vi "Generate Sound.vi"() -> ()   [LabVIEW 2017]
doc: "本VI说明了生成并播放正弦波、方波、锯齿波和三角波的方式。在连续播放时可更改生成波形的频率和类型。"
uses:
  <vilib>/sound2/lvsound2.llb/Sampling Mode.ctl
  <vilib>/sound2/lvsound2.llb/Sound Data Format.ctl
  <vilib>/sound2/lvsound2.llb/Sound Output Set Volume (Single).vi
  <vilib>/sound2/lvsound2.llb/Sound Output Write (DBL Single).vi
panel:
  in  "音量":dbl(slide)=50.0 scale=0.0..100.0
  out "生成声音":waveform(dbl)(graph)
  in  "频率":dbl=500.0
  in  "停止":bool
  in  "设备ID":u32
  # "概述：演示使用声音函数连续生成和播放正弦波形。\n操作步骤：\n1.指定设备ID的值。\n2. 运行VI。生成波形并将其发送至图形和扬声器。\n3.修改声音的频率和音量。\n4.单击停止按钮停止VI。"
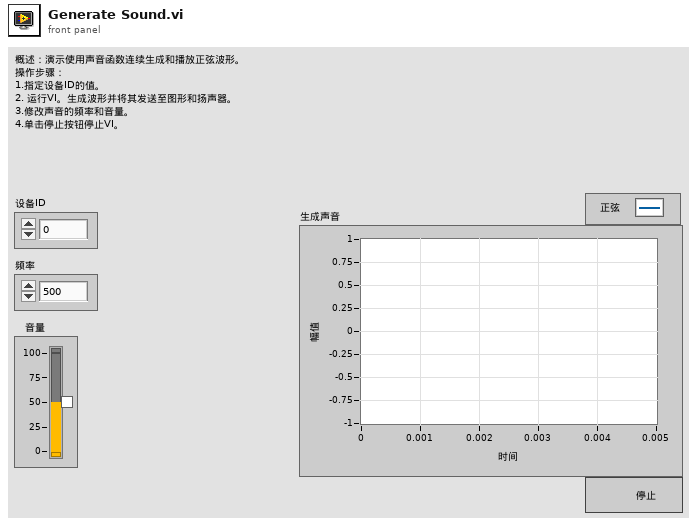
[diagram p1: front panel]
types:
  T1 = typedef "Sound Data Format.ctl" = cluster{"sample rate (S/s)":dbl, "number of channels":i32, "bits per sample":i32}
  T2 = typedef "Sampling Mode.ctl" = i32
  T3 = typedef "Sound Output Task ID.ctl" = u32
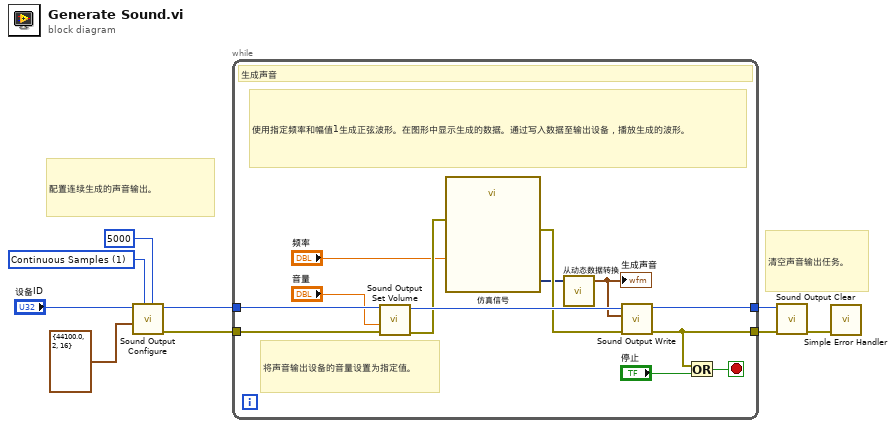
[diagram p0: block diagram]
diagram:
  w4 = T2 1 items=["Finite Samples", "Continuous Samples"] ("sample mode")
  # "配置连续生成的声音输出。"
  # "清空声音输出任务。"
  n1 = call <vilib>:"Sound Output Configure.vi"("number of samples/ch"=5000 ("Number of Samples/ch"), "sample mode"=w4, "sound format"=T1 {"sample rate (S/s)"=44100.0, "number of channels"=2, "bits per sample"=16} ("Sound Format"), "device ID"="设备ID") -> ("error out"=w9:errorcluster, "task ID"=w8:T3)  [unwired: 6 in]
  n2 = while {
    tunnel: w8 -> [w17]
    tunnel: [w22] -> w6
    tunnel: w9 -> [w19]
    tunnel: [w15] -> w7
    stop <- w20 stop-if-true
    # "将声音输出设备的音量设置为指定值。"
    # "使用指定频率和幅值1生成正弦波形。在图形中显示生成的数据。通过写入数据至输出设备，播放生成的波形。"
    # "生成声音"
    n3 = call-poly <vilib>:"Sound Output Set Volume.vi"("error in (no error)"=w19, "volume"="音量", "task ID"=w17) -> ("error out"=w13:errorcluster, "task ID out"=w18:T3)  [unwired: 7 in]
    n4 = call "仿真信号"("Frequency"="频率", "error in (no error)"=w13) -> ("Sine"=w11:dynamicdata, "error out"=w12:errorcluster)  [unwired: 12 in]
    n5 = call "从动态数据转换"("Dynamic Data Type"=w11) -> ("Waveform"=w14:waveform(dbl))  [unwired: 3 in]
    "生成声音" <- w14
    n6 = call-poly <vilib>:"Sound Output Write.vi"("error in (no error)"=w12, "data"=w14, "task ID"=w18) -> ("error out"=w15:errorcluster, "task ID out"=w22:T3)  [unwired: 7 in]
    n7 = Or(x=w15, y="停止") -> (x .or. y?=w20:bool)
  }
  n8 = call <vilib>:"Sound Output Clear.vi"("error in (no error)"=w7, "task ID"=w6) -> ("error out"=w2:errorcluster)  [unwired: 9 in]
  n9 = call <vilib>:"Simple Error Handler.vi"("error in (no error)"=w2) -> ()  [unwired: 4 in, 5 out]
